vi "GUI main.vi"() -> ()   [LabVIEW 2015]
panel:
  in  "obsticle location":i32[](array[numeric])=[20, 20]
  out "Map original":u16[][](array[ring])
  in  "stop":bool
  out "error out":errorcluster
  out "NSEW":dbl[](array[numeric])
  in  "error in (no error)":errorcluster
  in  "Start":bool
  out "Robot Direction":string
  out "Target Location":dbl[](array[numeric])
  out "DaNI location":dbl[](array[numeric])
  out "Map Display":u16[][](array[ring])
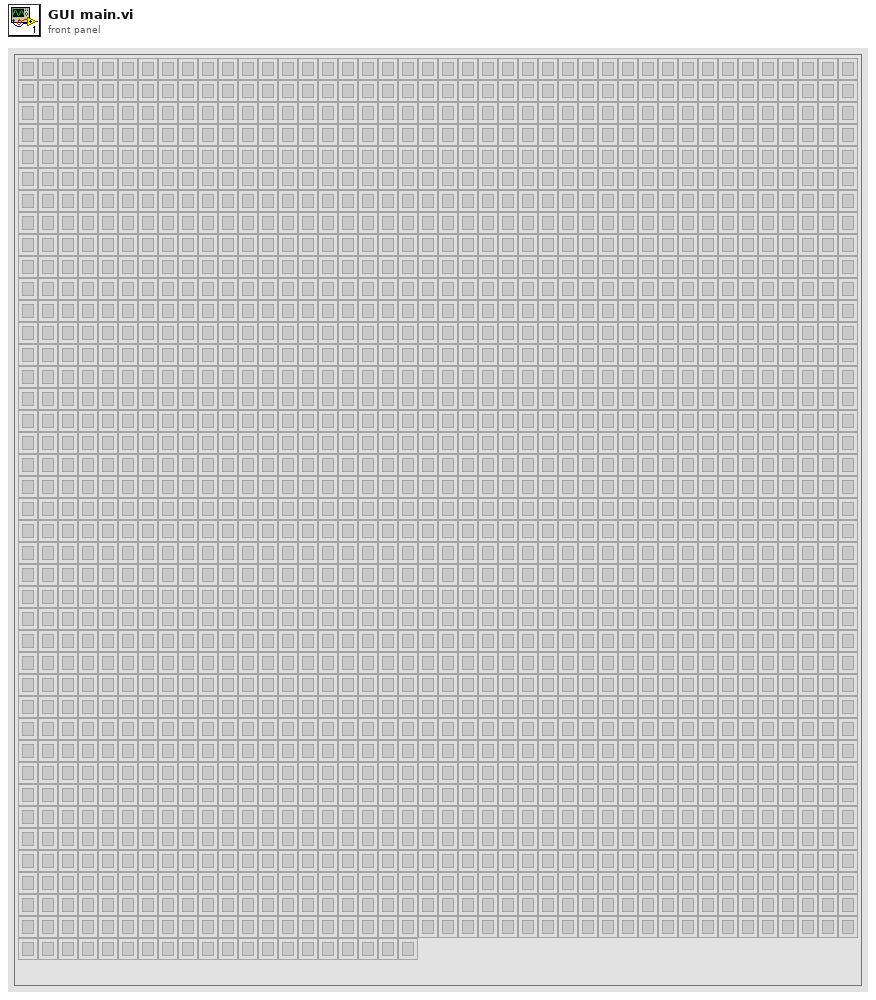
[diagram p1: front panel]
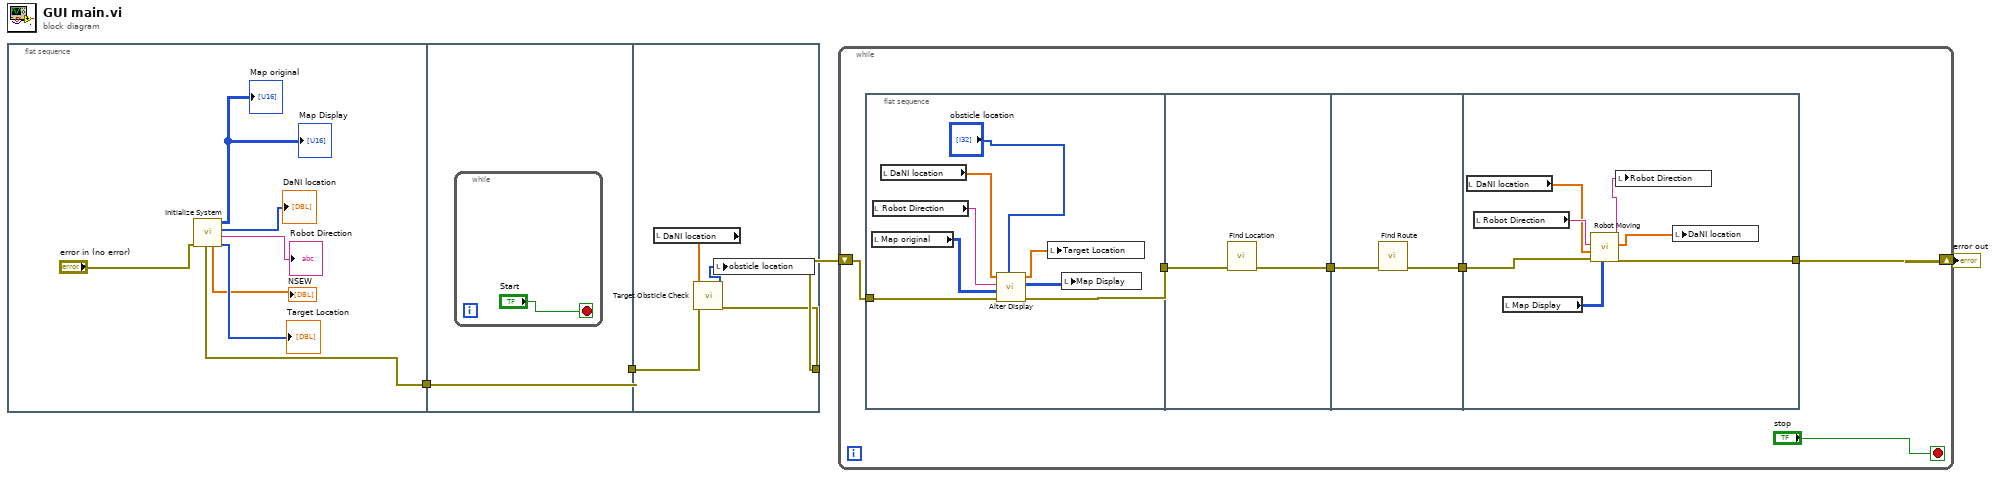
[diagram p0: block diagram]
diagram:
  n1 = flat-sequence {
    tunnel: [w6] -> w3
    tunnel: w3 -> [w12]
    tunnel: [w12] -> w1
    tunnel: [w16] -> w2
    tunnel: w1 -> [w17]
    frame #0 {
      n2 = call "Initialize System.vi"("error in (no error)"="error in (no error)") -> ("Target Location"=→"Target Location":i32[], "Direction"=→"Robot Direction":string, "Robot Location"=→"DaNI location":i32[], "Map"=→"Map Display" →"Map original":i32[][], "NSEW"=→"NSEW":dbl[], "error out"=w6:errorcluster)  [unwired: 5 in]
    }
    frame #1 {
      n3 = while {
        stop <- "Start" stop-if-true
      }
    }
    frame #2 {
      n4 = local read "DaNI location"() -> (w15:dbl[])
      n5 = call "Target Obsticle Check.vi"("error in (no error)"=w17, "DaNI location"=w15) -> ("error out"=w16:errorcluster, "obsticle location"=w14:i32[])  [unwired: 8 in]
      n6 = local write "obsticle location"(w14) -> ()
    }
  }
  n7 = while {
    shift-right: [w20] -> w4
    shift-left: w2 -> [w18]
    stop <- "stop" stop-if-true
    n8 = flat-sequence {
      tunnel: [w31] -> w23
      tunnel: w18 -> [w24]
      tunnel: w23 -> [w33]
      tunnel: [w32] -> w22
      tunnel: [w35] -> w21
      tunnel: w22 -> [w34]
      tunnel: [w42] -> w20
      tunnel: w21 -> [w41]
      frame #0 {
        n9 = local read "Map original"() -> (w30:u16[][])
        n10 = local read "Robot Direction"() -> (w28:string)
        n11 = local read "DaNI location"() -> (w29:dbl[])
        n12 = call "Alter Display.vi"("obsticle location"="obsticle location", "error in (no error)"=w24, "Display Map"=w30, "robot direction"=w28, "robot location"=w29) -> ("error out"=w31:errorcluster, "Map"=w26:u16[][], "target location"=w27:dbl[])  [unwired: 4 in]
        n13 = local write "Target Location"(w27) -> ()
        n14 = local write "Map Display"(w26) -> ()
      }
      frame #1 {
        n15 = call "Find Location.vi"("error in (no error)"=w33) -> ("error out"=w32:errorcluster)  [unwired: 10 in]
      }
      frame #2 {
        n16 = call "Find Route.vi"("error in (no error)"=w34) -> ("error out"=w35:errorcluster)  [unwired: 10 in]
      }
      frame #3 {
        n17 = local read "DaNI location"() -> (w39:dbl[])
        n18 = local read "Robot Direction"() -> (w40:string)
        n19 = local read "Map Display"() -> (w38:u16[][])
        n20 = call "Robot Moving.vi"("Priority level array"=w38, "error in (no error)"=w41, "location"=w39, "direction"=w40) -> ("error out"=w42:errorcluster, "new location"=w37:dbl[], "new direction"=w36:string)  [unwired: 5 in]
        n21 = local write "Robot Direction"(w36) -> ()
        n22 = local write "DaNI location"(w37) -> ()
      }
    }
  }
  "error out" <- w4
